vi "Switch-DMM RT Driver VI.vi"(7 "Operation":T1, 11 "Device Reference in":T2 format="%.0x") -> (0 "Error Code":i32)   [LabVIEW 2011, in "Switch-DMM Custom Device.lvlib"]
uses:
  Switch-DMM Custom Device.lvlib
  <vilib>/NI Veristand/Custom Device API/Custom Device Item Ref.ctl
  <vilib>/NI Veristand/Custom Device API/Hardware Interface Driver VI Operation.ctl
  Controls/RT Data.ctl
  Controls/Channels.ctl
  Controls/Single Channel.ctl
  <vilib>/NI Veristand/Custom Device API/Data Reference.ctl
  Controls/Block Channels.ctl
  <vilib>/NI Veristand/Custom Device API/Block Data Reference.ctl
  Controls/Communication.ctl
  Controls/Async Status.ctl
  Controls/Async State.ctl
  Controls/Async Command.ctl
  Controls/Async Events.ctl
  <vilib>/NI Veristand/Custom Device API/Custom Device API.lvlib
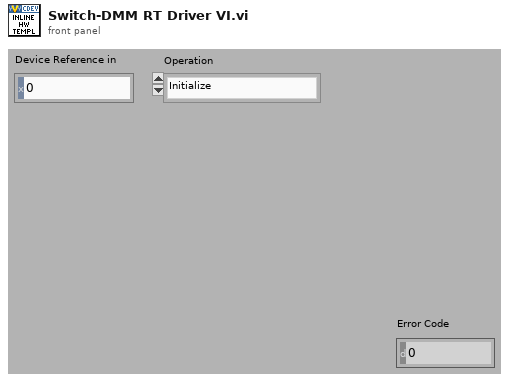
[diagram p1: front panel]
types:
  T1 = typedef "Custom Device API.lvlib/Hardware Interface Driver VI Operation.ctl" = enum16{"Initialize", "Start", "Read Data from HW", "Write Data to HW", "Close"}
  T2 = typedef "Custom Device API.lvlib/Custom Device Item Ref.ctl" = u64
  T3 = typedef "Switch-DMM Custom Device.lvlib/RT Data.ctl" = cluster{"Channels":T4, "Communication":T9}
  T4 = typedef "Switch-DMM Custom Device.lvlib/Channels.ctl" = cluster{"Mode":T5, "Read Volt":T5, "Current":T7, "Voltage":T7}
  T5 = typedef "Switch-DMM Custom Device.lvlib/Single Channel.ctl" = cluster{"Ref":T6, "Value":bool}
  T6 = typedef "Custom Device API.lvlib/Data Reference.ctl" = i32
  T7 = typedef "Switch-DMM Custom Device.lvlib/Block Channels.ctl" = cluster{"Ref":T8[], "Value":dbl[]}
  T8 = typedef "Custom Device API.lvlib/Block Data Reference.ctl" = cluster{"Data Reference":T6, "Offset":i32, "Length":i32}
  T9 = typedef "Switch-DMM Custom Device.lvlib/Communication.ctl" = cluster{"Status Q":refnum<queue>, "Command Q":refnum<queue>, "Voltage FIFO":refnum<k33>, "Voltage Buffer":dbl[], "Current FIFO":refnum<k33>, "Current Buffer":dbl[], "Async Events":refnum<queue>}
  T10 = typedef "Switch-DMM Custom Device.lvlib/Async State.ctl" = enum16{"Not running", "Initializing", "Waiting on start cmd", "Running", "Stopped"}
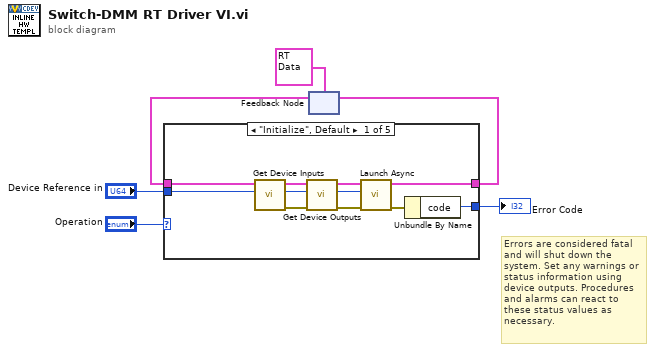
[diagram p0: block diagram]
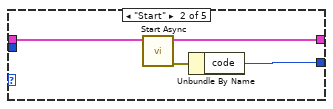
[diagram p2: hidden frame]
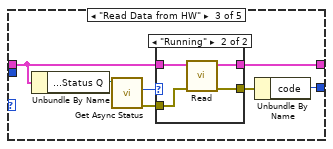
[diagram p3: hidden frame]
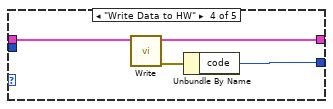
[diagram p5: hidden frame]
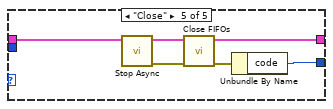
[diagram p6: hidden frame]
diagram:
  # "Errors are considered fatal and will shut down the system. Set any warnings or status information using device outputs. Procedures and alarms can react to these status values as necessary."
  n1 = feedback #1(T3 {"Channels"={"Mode"={"Ref"=0, "Value"=FALSE}, "Read Volt"={"Ref"=0, "Value"=FALSE}, "Current"={"Ref"=[], "Value"=[]}, "Voltage"={"Ref"=[], "Value"=[]}}, "Communication"={"Status Q"=refnum, "Command Q"=refnum, "Voltage FIFO"=refnum, "Voltage Buffer"=[], "Current FIFO"=refnum, "Current Buffer"=[], "Async Events"=refnum}} ("RT Data")) -> (w4:T3)
  n2 = case shown="\"Initialize\", Default" "Operation" {
    tunnel: [w7 w18 w26 w37 w39] -> w5
    tunnel: w4 -> [w9 w19 w27 w38 w42]
    tunnel: "Device Reference in" -> [w8 _ _ _ _]
    tunnel: [w17 w20 w28 w36 w41] -> w2
    frame "Initialize", Default {
      n3 = call "Get Device Inputs.vi"("Device Reference in"=w8, "RT Data in"=w9) -> ("error out"=w15:errorcluster, "Device Ref out"=w14:T2, "RT Data out"=w13:T3)  [unwired: 7 in]
      n4 = call "Get Device Outputs.vi"("error in (no error)"=w15, "Device Reference in"=w14, "RT Data in"=w13) -> ("error out"=w11:errorcluster, "Device Ref out"=w10:T2, "RT Data out"=w12:T3)  [unwired: 6 in]
      n5 = call "Launch Async.vi"("error in (no error)"=w11, "Device Ref in"=w10, "RT Data in"=w12) -> ("error out"=w16:errorcluster, "RT Data out"=w7:T3)  [unwired: 6 in, 1 out]
      n6 = Unbundle By Name(w16) -> ("code"=w17:i32)
    }
    frame "Start" {
      n7 = call "Start Async.vi"("RT Data in"=w19) -> ("error out"=w21:errorcluster, "RT Data out"=w18:T3)  [unwired: 9 in]
      n8 = Unbundle By Name(w21) -> ("code"=w20:i32)
    }
    frame "Read Data from HW" {
      n9 = Unbundle By Name(w27) -> ("Communication.Status Q"=w25:refnum<queue>)
      n10 = call "Get Async Status.vi"("queue in"=w25) -> ("error out"=w23:errorcluster, "State"=w24:T10)  [unwired: 8 in, 1 out]
      n11 = case shown="\"Running\"" w24 {
        tunnel: w23 -> [w30 w34]
        tunnel: [w30 w32] -> w22
        tunnel: w27 -> [w29 w33]
        tunnel: [w29 w31] -> w26
        frame "Not running", Default {
        }
        frame "Running" {
          n12 = call "Read.vi"("error in (no error)"=w34, "RT Data in"=w33) -> ("error out"=w32:errorcluster, "RT Data out"=w31:T3)  [unwired: 8 in]
        }
      }
      n13 = Unbundle By Name(w22) -> ("code"=w28:i32)
    }
    frame "Write Data to HW" {
      n14 = call "Write.vi"("RT Data in"=w38) -> ("error out"=w35:errorcluster, "RT Data out"=w37:T3)  [unwired: 9 in]
      n15 = Unbundle By Name(w35) -> ("code"=w36:i32)
    }
    frame "Close" {
      n16 = call "Stop Async.vi"("RT Data in"=w42) -> ("error out"=w43:errorcluster, "RT Data out"=w40:T3)  [unwired: 9 in]
      n17 = call "Close FIFOs.vi"("error in (no error)"=w43, "RT Data in"=w40) -> ("error out"=w44:errorcluster, "RT Data out"=w39:T3)  [unwired: 8 in]
      n18 = Unbundle By Name(w44) -> ("code"=w41:i32)
    }
  }
  "Error Code" <- w2
  n19 = feedback-in #1(w5) -> ()
